vi "TempRead (SubVI).vi"(8 "error in (no error)":errorcluster, 11 "Refnum in":refnum<k21>) -> (0 "error out":errorcluster, 1 "Temp (F)":dbl, 2 "Resistance":dbl format="%0.2f", 3 "Refnum out":refnum<k21>)   [LabVIEW 2020]
uses:
  <vilib>/DAQmx/read.llb/DAQmx Read (Analog DBL 1Chan 1Samp).vi
  <vilib>/DAQmx/miscellaneous.llb/DAQmx Fill In Error Info.vi
  <vilib>/express/express arith-compare/Formula/XNode/ExpressFormulaBlockNode.xnode
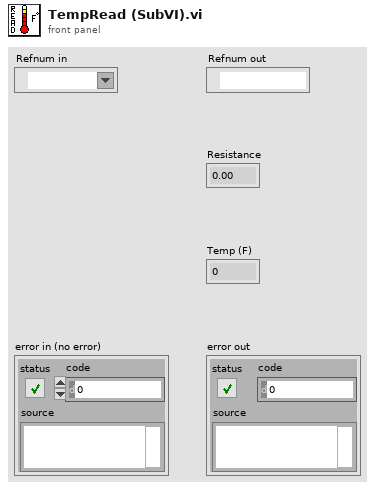
[diagram p1: front panel]
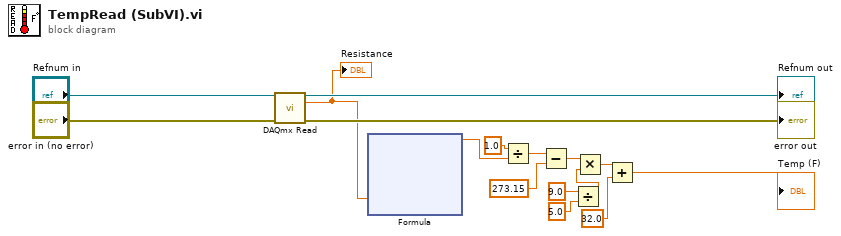
[diagram p0: block diagram]
diagram:
  n1 = call-poly <vilib>:"DAQmx Read.vi"("task/channels in"="Refnum in", "error in"="error in (no error)") -> ("task out"=→"Refnum out":refnum<k21>, "data"=w1:dbl, "error out"=→"error out":errorcluster)  [unwired: 11 in]
  "Resistance" <- w1
  n2 = xnode "Formula"("X1"=w1) -> ("Result"=w2:dbl)  [unwired: 1 in, 1 out]
  n3 = Divide(x=1.0, y=w2) -> (x/y=w4:dbl)
  n4 = Subtract(x=w4, y=273.15) -> (x-y=w8:dbl)
  n5 = Divide(x=9.0, y=5.0) -> (x/y=w9:dbl)
  n6 = Multiply(x=w8, y=w9) -> (x*y=w10:dbl)
  n7 = Add(x=w10, y=32.0) -> (x+y=→"Temp (F)":dbl)
